vi "Properties to Tree Array.vi"(7 "Action":T1, 10 "Tree Type":enum16{"Main", "Write", "Read"}(ring), 11 "Properties for Tree":T3(array[cluster])) -> (3 "Tree Arr":T2(array[cluster]))   [LabVIEW 2023]
doc: "Convert property info to array for tree display, including setting glyph.\n\nDo not set indents for R/W trees here, wait until after filtering."
uses:
  controls/action enum.ctl
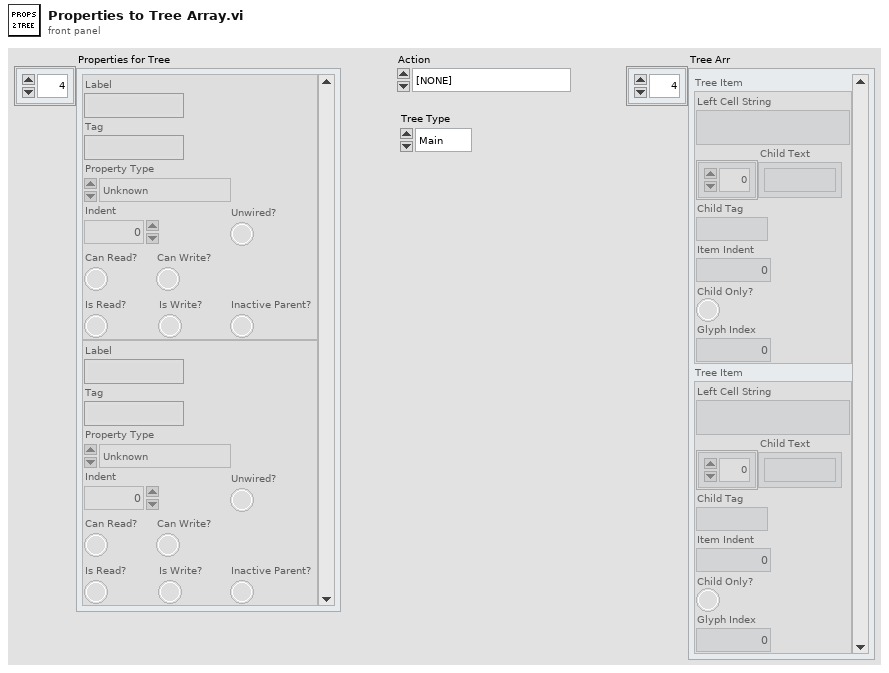
[diagram p1: front panel]
types:
  T1 = typedef "action enum.ctl" = enum16{"[NONE]", "Wire Bundle", "Wire Unbundle", "Terminal Unbundle", "Terminal Bundle", "Bundler Move Up", "Bundler Move Down", "Bundler Insert", "Bundler Remove", "Bundler Remove Unwired", "Bundler Rearrange", "In Place Insert", "In Place Remove", "In Place Remove Unwired", "In Place Rearrange", "Wire Properties", "Wire Method", "Terminal Properties", "Terminal Method", "Property Move Up", "Property Move Down", "Properties Insert", "Properties Remove", "Properties Remove Unwired", "Properties Rearrange", "Method Change", "Class for Constant", "Class For Control", "Class For Node", "Class Name to Clipboard"}
  T2 = cluster{"Left Cell String":string, "Child Text":string[], "Child Tag":string, "Item Indent":i32, "Child Only?":bool, "Glyph Index":i32}[]
  T3 = cluster{"Label":string, "Tag":string, "Property Type":enum16{"Unknown", "Base", "Scripting", "Private", "Deprecated", "None", "Divider"}, "Indent":u16, "Can Read?":bool, "Can Write?":bool, "Is Read?":bool, "Is Write?":bool, "Inactive Parent?":bool, "Unwired?":bool}[]
  T4 = cluster{"Left Cell String":string, "Child Text":string[], "Child Tag":string, "Item Indent":i32, "Child Only?":bool, "Glyph Index":i32}
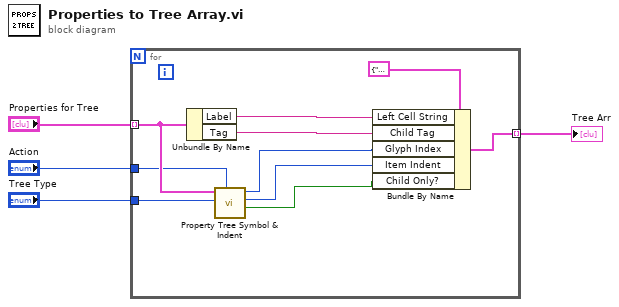
[diagram p0: block diagram]
diagram:
  n1 = for {
    tunnel: "Properties for Tree" -> [w10] mode=indexing
    tunnel: [w14] -> w3 mode=indexing
    tunnel: "Action" -> [w7]
    tunnel: "Tree Type" -> [w6]
    n2 = Unbundle By Name(w10) -> ("Label"=w12:string, "Tag"=w13:string)
    n3 = call "Property Tree Symbol & Indent.vi"("Action"=w7, "Tree Type"=w6, "Property Info"=w10) -> ("Child Only?"=w5:bool, "Indent"=w8:u16, "Symbol"=w9:i32)  [unwired: 6 in]
    n4 = Bundle By Name(cluster=T4 {"Left Cell String"="", "Child Text"=[], "Child Tag"="", "Item Indent"=0, "Child Only?"=FALSE, "Glyph Index"=0} ("Tree Item"), "Left Cell String"=w12, "Child Tag"=w13, "Glyph Index"=w9, "Item Indent"=w8, "Child Only?"=w5) -> (w14:T4)
  }
  "Tree Arr" <- w3
